vi "Format LogRecord.vi"(8 "error in":errorcluster, 10 "LogRecord":refnum<class "LogRecord.lvclass">, 11 "LokiJsonFormatter in":refnum<class "LokiJsonFormatter.lvclass">) -> (0 "error out":errorcluster, 2 "LogLine":string)   [LabVIEW 2019, in "hse-logger.lvlib" / "LokiJsonFormatter.lvclass"]
doc: "Format the Log Record with the formatter class to retrieve a JSON object that is being sent to loki by the handler."
uses:
  LokiJsonFormatter.lvclass
  LogRecord/LogRecord.lvclass
  LokiJsonFormatter.lvclass/LokiJsonFormatter.ctl
panel:
  # "Connector Pane"
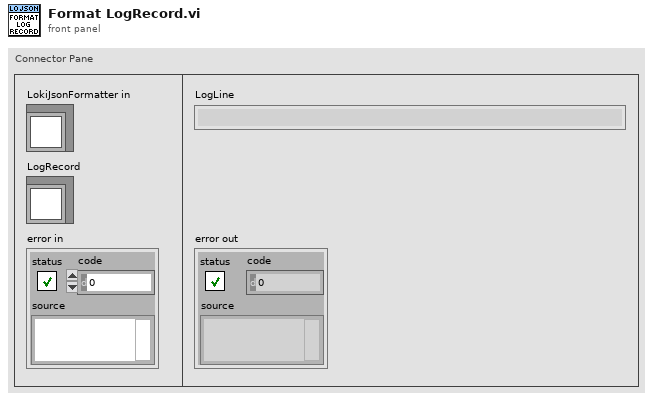
[diagram p1: front panel]
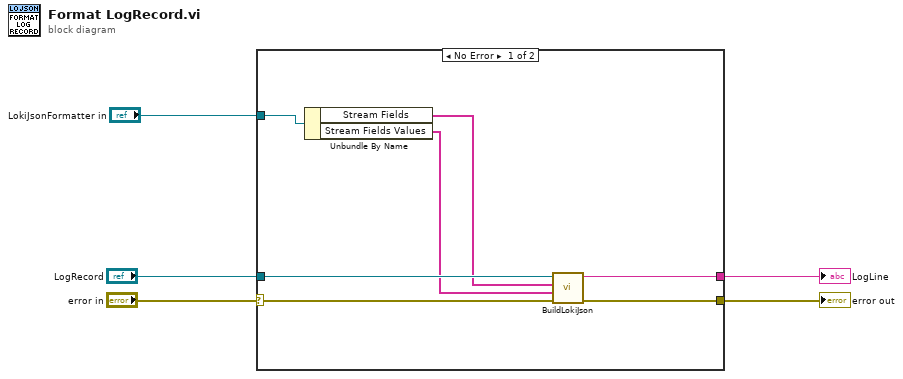
[diagram p0: block diagram]
diagram:
  n1 = case shown="No Error" "error in" {
    selector: "error in" -> [w11 w13]
    tunnel: [w10 w13] -> w2
    tunnel: "LogRecord" -> [w9 _]
    tunnel: "LokiJsonFormatter in" -> [w12 _]
    tunnel: [w6 _] -> w1
    frame No Error {
      n2 = Unbundle By Name(w12) -> ("Stream Fields"=w8:string[], "Stream Fields Values"=w7:string[])
      n3 = call "BuildLokiJson.vi"("error in (no error)"=w11, "Stream Fields Values"=w7, "Stream Fields"=w8, "LogRecord"=w9) -> ("error out"=w10:errorcluster, "<JSON> out"=w6:string)  [unwired: 6 in]
    }
    frame Error {
    }
  }
  "error out" <- w2
  "LogLine" <- w1
